vi "NanoStageGetPositions.vi"(7 "error in (no error)":errorcluster, 10 "Config In":T1) -> (0 "error out":errorcluster, 2 "Positions":cluster{"Time":dbl, "x":dbl, "y":dbl, "z":dbl}, 3 "Config Out":T1)   [LabVIEW 2019, in "Acquisition.lvlib"]
doc: "Generates sample waveforms according to the signal type in the HW Config input."
uses:
  Acquisition.lvlib
  Settings/Settings.ctl
  HardwareAdapter/Support/Hardware Configuration.ctl
  HardwareAdapter/Support/Camera Configuration.ctl
  E:/DevHardSoftware/MMicroscopy/HardwareAdapter/Camera/Dependencies/PVCamNET.dll
  HardwareAdapter/Camera/Dependencies/PVCamNET.dll
  <vilib>/userdefined/High Color/IMAQdx.ctl
  Logging/Logging Configuration.ctl
  controls/UI Configuration.ctl
  <vilib>/numeric/Random Number (Range) U64.vi
  <vilib>/numeric/sub_Random U32.vi
  Logging/Logging.lvlib
  Settings/Settings.lvlib
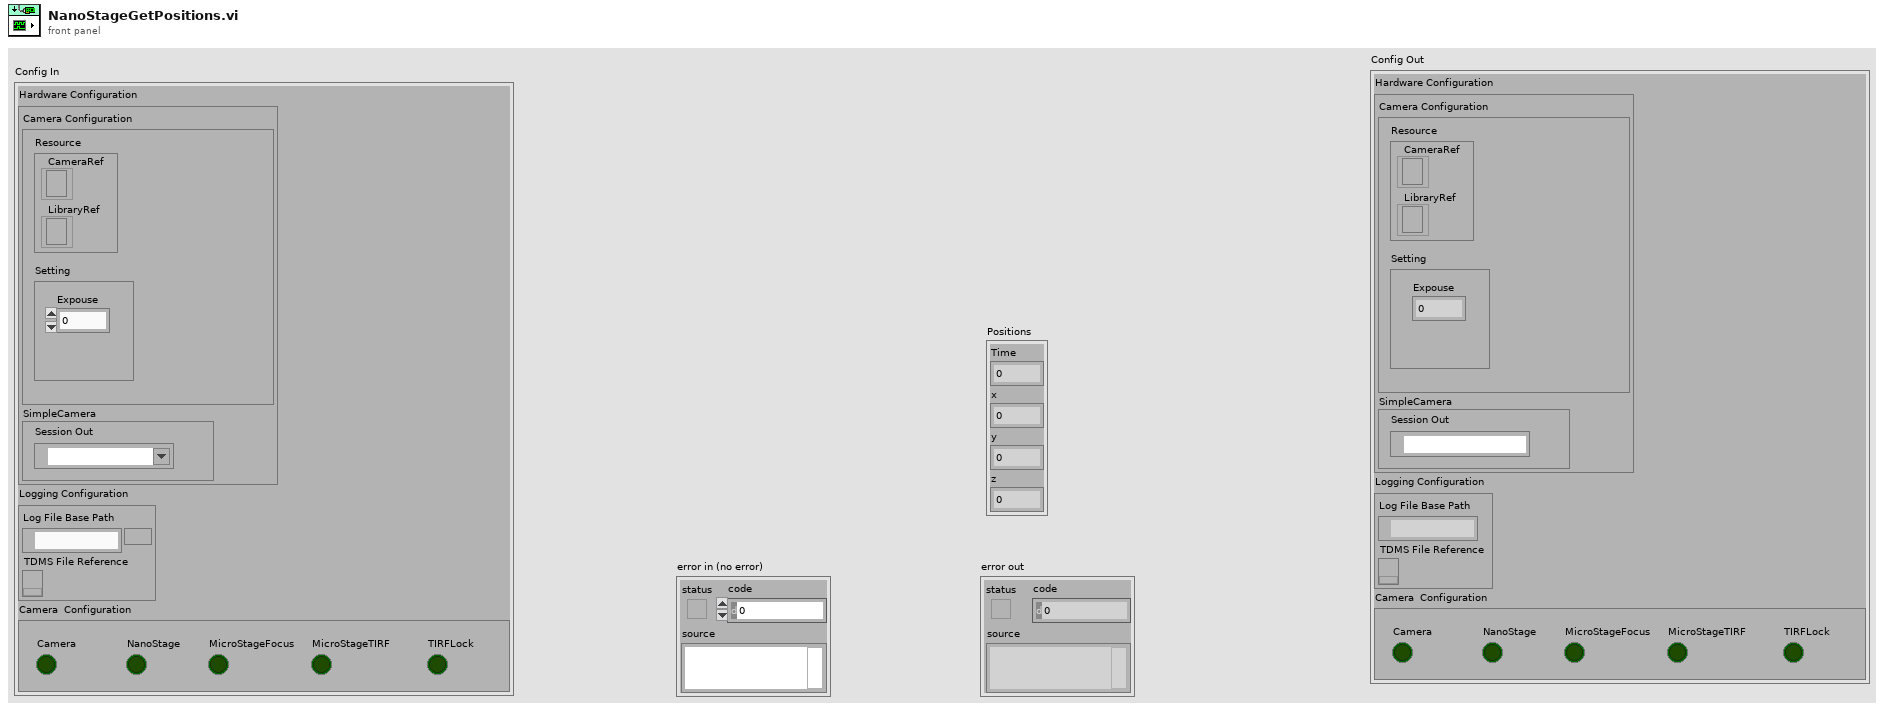
[diagram p1: front panel]
types:
  T1 = typedef "Settings.lvlib/Settings.ctl" = cluster{"Hardware Configuration":T2, "Logging Configuration":T5, "UI Configuration":T6}
  T2 = typedef "Hardware Configuration.ctl" = cluster{"Camera Configuration":T3, "SimpleCamera":cluster{"Session Out":T4}}
  T3 = typedef "Camera Configuration.ctl" = cluster{"Resource":cluster{"CameraRef":refnum<k24>, "LibraryRef":refnum<k24>}, "Setting":cluster{"Expouse":dbl}}
  T4 = typedef "IMAQdx.ctl" = refnum<k21>
  T5 = typedef "Logging.lvlib/Logging Configuration.ctl" = cluster{"Log File Base Path":path, "TDMS File Reference":refnum<k34>}
  T6 = typedef "UI Configuration.ctl" = cluster{"Camera":bool, "NanoStage":bool, "MicroStageFocus":bool, "MicroStageTIRF":bool, "TIRFLock":bool}
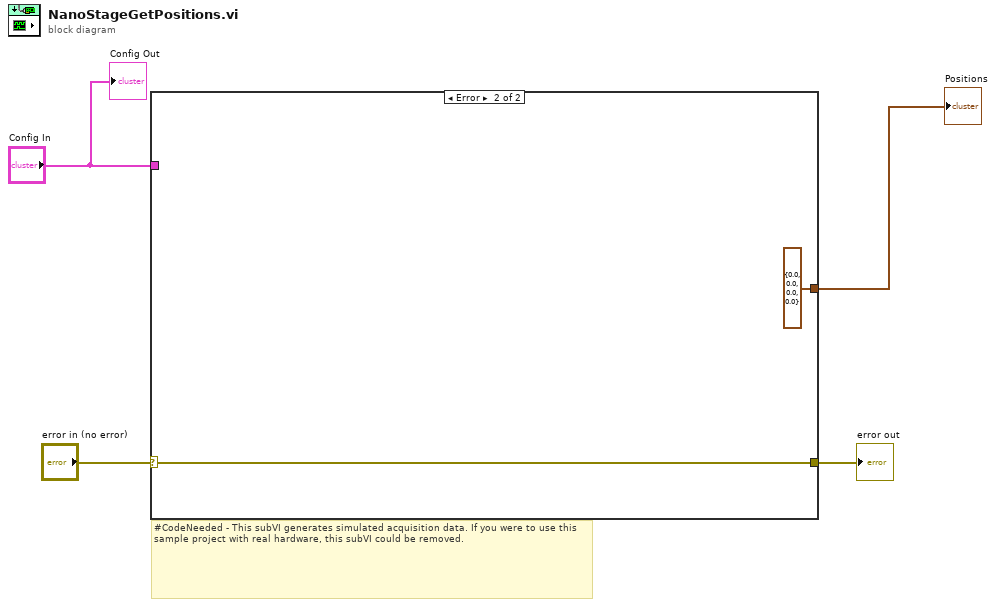
[diagram p0: block diagram]
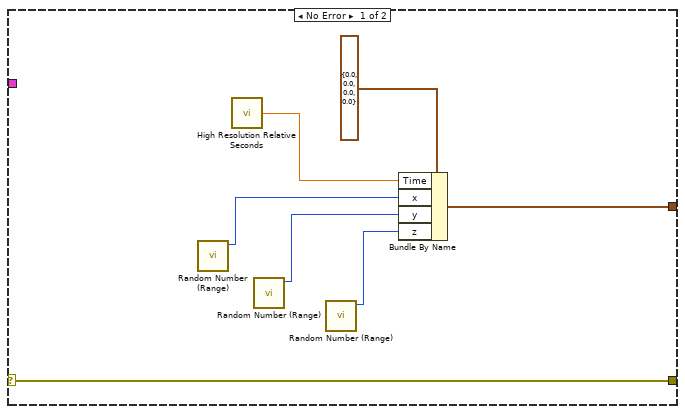
[diagram p2: hidden frame]
diagram:
  # "#CodeNeeded - This subVI generates simulated acquisition data. If you were to use this sample project with real hardware, this subVI could be removed."
  n1 = case shown="Error" "error in (no error)" {
    selector: "error in (no error)" -> [w11 w13]
    tunnel: [w11 w13] -> w3
    tunnel: "Config In" -> [_ _]
    tunnel: [w5 cluster{"Time":dbl, "x":dbl, "y":dbl, "z":dbl} {"Time"=0.0, "x"=0.0, "y"=0.0, "z"=0.0} ("RawImage")] -> w1
    frame No Error {
      n2 = call-poly <vilib>:"Random Number (Range).vi"() -> ("number"=w8:u64)  [unwired: 11 in]
      n3 = call <vilib>:"High Resolution Relative Seconds.vi"() -> ("relative seconds"=w9:dbl)
      n4 = call-poly <vilib>:"Random Number (Range).vi"() -> ("number"=w7:u64)  [unwired: 11 in]
      n5 = call-poly <vilib>:"Random Number (Range).vi"() -> ("number"=w6:u64)  [unwired: 11 in]
      n6 = Bundle By Name(cluster=cluster{"Time":dbl, "x":dbl, "y":dbl, "z":dbl} {"Time"=0.0, "x"=0.0, "y"=0.0, "z"=0.0} ("RawImage"), "Time"=w9, "x"=w8, "y"=w7, "z"=w6) -> (w5:cluster{"Time":dbl, "x":dbl, "y":dbl, "z":dbl})
    }
    frame Error {
    }
  }
  "error out" <- w3
  "Positions" <- w1
  "Config Out" <- "Config In"
